vi "Configure Source (Limit).vi"(0 "VISA resource name":refnum<visa-resource-name>, 1 "Current Limit (0.1 A)":dbl=0.1, 2 "Power Limit (20 W)":dbl=20.0, 5 "Source Measure Unit Channel (0: Channel A)":i32(ring) items=["Channel A", "Channel B"], 7 "Limit Type (1: Voltage)":i32(ring)=1 items=["Current", "Voltage", "Power"], 11 "error in (no error)":errorcluster, 12 "Voltage Limit (20 V)":dbl=20.0) -> (4 "VISA resource name out":refnum<visa-resource-name>, 15 "error out":errorcluster)   [LabVIEW 2020, in "Keithley 2600 Series.lvlib"]
doc: "Configures the compliance limits."
uses:
  Keithley 2600 Series.lvlib
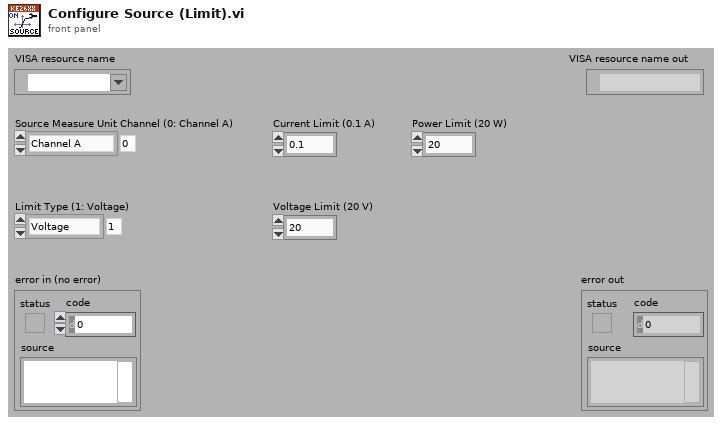
[diagram p1: front panel]
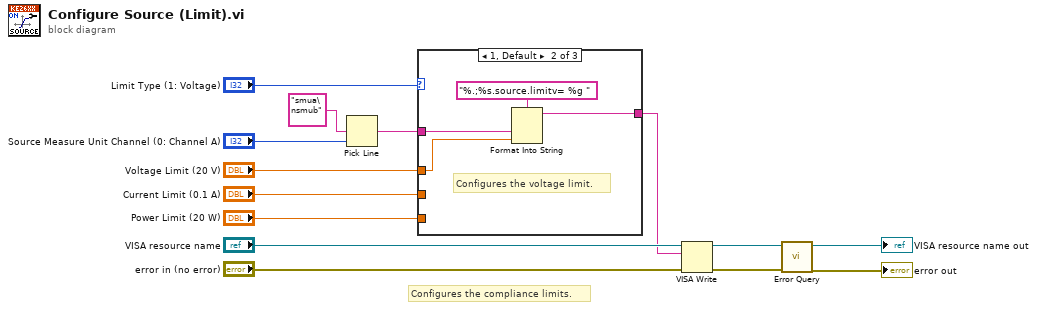
[diagram p0: block diagram]
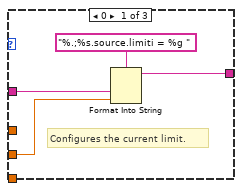
[diagram p2: hidden frame]
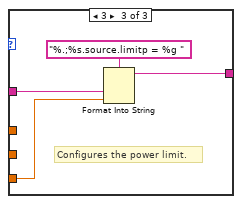
[diagram p3: hidden frame]
diagram:
  # "Configures the compliance limits."
  n1 = Pick Line(multi-line string="smua\nsmub", line index="Source Measure Unit Channel (0: Channel A)") -> (output string=w5:string)  [unwired: 1 in]
  n2 = case shown="1, Default" "Limit Type (1: Voltage)" {
    tunnel: w5 -> [w17 w21 w25]
    tunnel: "Voltage Limit (20 V)" -> [_ w19 _]
    tunnel: [w16 w20 w24] -> w3
    tunnel: "Current Limit (0.1 A)" -> [w15 _ _]
    tunnel: "Power Limit (20 W)" -> [_ _ w23]
    frame 0 {
      # "Configures the current limit."
      n3 = Format Into String(format string="%.;%s.source.limiti = %g ", w17, w15) -> (resulting string=w16:string)  [unwired: 2 in, 1 out]
    }
    frame 1, Default {
      # "Configures the voltage limit."
      n4 = Format Into String(format string="%.;%s.source.limitv= %g ", w21, w19) -> (resulting string=w20:string)  [unwired: 2 in, 1 out]
    }
    frame 3 {
      # "Configures the power limit."
      n5 = Format Into String(format string="%.;%s.source.limitp = %g ", w25, w23) -> (resulting string=w24:string)  [unwired: 2 in, 1 out]
    }
  }
  n6 = VISA Write(VISA resource name="VISA resource name", write buffer=w3, error in (no error)="error in (no error)") -> (VISA resource name out=w12:refnum<visa-resource-name>, error out=w11:errorcluster)  [unwired: 1 out]
  n7 = call "Error Query.vi"("error in (no error)"=w11, "VISA resource name"=w12) -> ("error out"=→"error out":errorcluster, "VISA resource name out"=→"VISA resource name out":refnum<visa-resource-name>)  [unwired: 6 in, 2 out]
